vi "Program list Selection.vi"(8 "error in":errorcluster, 9 "FeedBack Channel":string[](array[string])=["fgdgfvcbc", "vnfhgjkn", "21354682"], 10 "Filepath":path=path "D:/My Project/2019-2020/Magnetic Mareli UM/MM_UM/Project Setup/data/program seq/Program_280A.bin", 11 "vi referenceIn":refnum<vi>) -> (0 "error out":errorcluster, 1 "Exit":bool, 2 "String":string, 3 "vi reference Out":refnum<vi>)   [LabVIEW 2015]
uses:
  Control Button/Exit.ctl
  Control Button/next.ctl
  Control Button/Control 11.ctl
  Galobal variable_TI.vi
  <vilib>/addons/database/Connection.llb/DB Tools Open Connec (String).vi
  <vilib>/addons/database/_DB Variant To Data/Database Variant To Data.xnode
  <vilib>/addons/database/NI_Database_API.lvlib
panel:
  out "error out 2":errorcluster
  out "String 2":string
  in  "Next":T1
  in  "Exit":T2
  in  "Program List":string(combo)
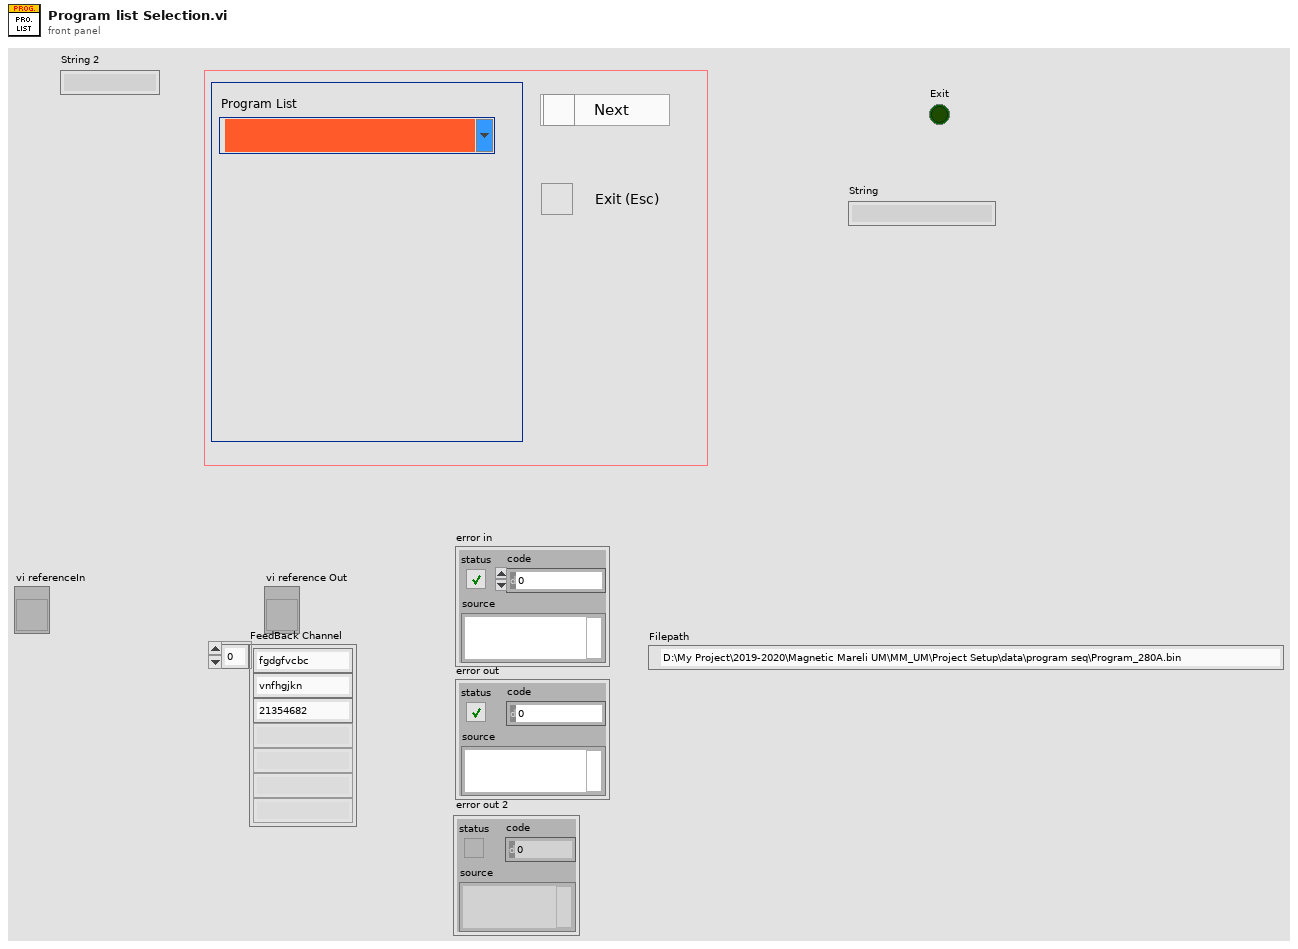
[diagram p1: front panel]
types:
  T1 = typedef "next.ctl" = bool
  T2 = typedef "Exit.ctl" = bool
  T3 = typedef "Control 11.ctl" = dbl
  T4 = enum32{"Invalid", "Standard", "Closed", "Hidden", "Minimized", "Maximized"}
  T5 = typedef "NI_Database_API.lvlib/Conn ObjectReference.ctl" = refnum<k1>
  T6 = cluster{"LVDT1Max AI0":dbl, "LVDT1Min AI0":dbl, "LVDT2Max AI1":dbl, "LVDT2Min AI1":dbl, "LVDT3Max AI2":dbl, "LVDT3Min AI2":dbl, "LVDT4Max AI3":dbl, "LVDT4Min AI3":dbl, "Model":string, "MIC Code":string}
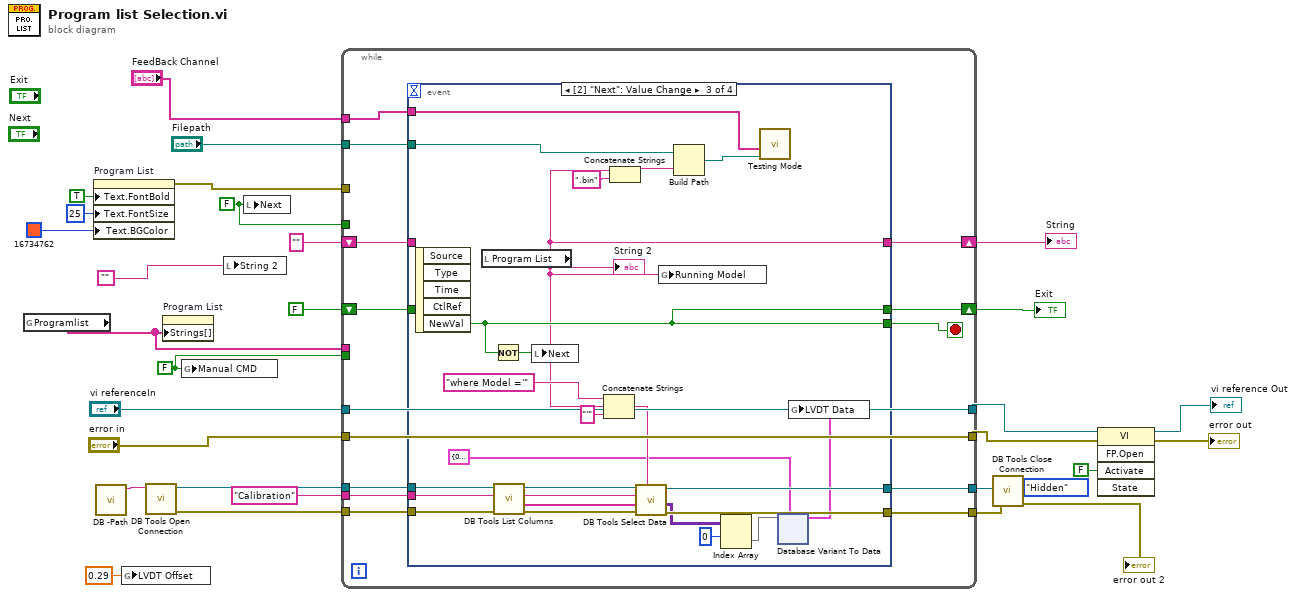
[diagram p0: block diagram]
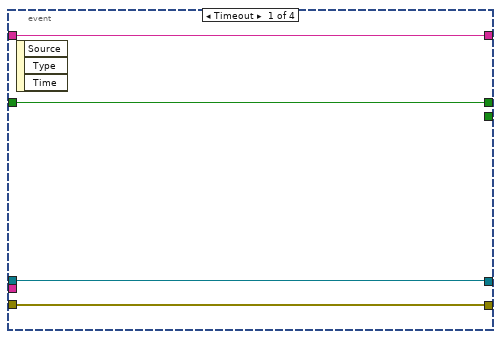
[diagram p2: hidden frame]
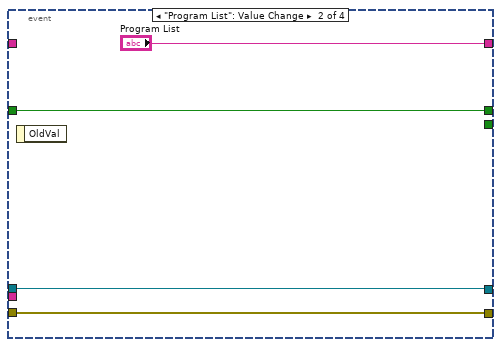
[diagram p3: hidden frame]
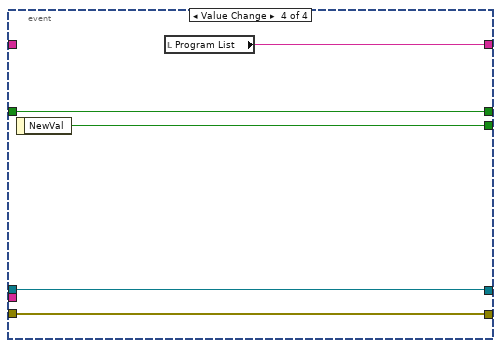
[diagram p4: hidden frame]
diagram:
  (unwired) T4."Hidden" ("State")
  w18 = FALSE ("Manual CMD")
  w19 = FALSE ("Next")
  n1 = global read "Galobal variable_TI.vi" "Programlist"() -> (w25:string[])
  n2 = property on="Program List" class="CmbBox"("Text.FontBold"=TRUE ("Text.Font:Bold"), "Text.FontSize"=u32 25 ("Text.Font:Size"), "Text.BGColor"=u32 16734762 ("Color Box")) -> (error out=w22:errorcluster)  [unwired: 2 in, 1 out]
  n3 = call "DB -Path.vi"() -> ("String"=w8:string)  [unwired: 11 in]
  n4 = global write "Galobal variable_TI.vi" "LVDT Offset"(T3 0.29 ("LVDT Offset")) -> ()
  n5 = call-poly <vilib>:"DB Tools Open Connection.vi"("connection information"=w8) -> ("error out"=w6:errorcluster, "connection reference"=w7:T5)  [unwired: 7 in]
  n6 = property on="Program List" class="CmbBox"("Strings[]"=w25) -> ()  [unwired: 2 in, 2 out]
  n7 = global write "Galobal variable_TI.vi" "Manual CMD"(w18) -> ()
  n8 = local write "String 2"("") -> ()
  n9 = local write "Next"(w19) -> ()
  n10 = while {
    shift-right: [w43] -> w29
    shift-left: "" ("Combo Box") -> [w42]
    shift-right: [w40] -> w26
    shift-left: T2 FALSE ("NewVal") -> [w39]
    tunnel: w25 -> [_]
    tunnel: w22 -> [_]
    tunnel: w19 -> [_]
    tunnel: w18 -> [_]
    tunnel: "vi referenceIn" -> [w38]
    tunnel: [w38] -> w12
    tunnel: "error in" -> [w37]
    tunnel: [w37] -> w11
    tunnel: "Filepath" -> [w36]
    tunnel: "FeedBack Channel" -> [w35]
    tunnel: w7 -> [w34]
    tunnel: w6 -> [w33]
    tunnel: "Calibration" ("table") -> [w32]
    tunnel: [w31] -> w4
    tunnel: [w30] -> w3
    stop <- w41 stop-if-true
    n11 = event shown="[2] \"Next\": Value Change" {
      selector: _ -> [_ _ _ _]
      dyn-events: _ -> [_ _ _ _]
      timeout: _ -> [_ _ _ _]
      tunnel: [w47 "Program List" w60 w393] -> w43
      tunnel: w42 -> [w47 _ _ _]
      tunnel: [_ _ w70 w394] -> w41
      tunnel: [w46 w50 w70 w392] -> w40
      tunnel: w39 -> [w46 w50 _ w392]
      tunnel: w36 -> [_ _ w73 _]
      tunnel: w35 -> [_ _ w71 _]
      tunnel: w34 -> [w45 w49 w66 w391]
      tunnel: w33 -> [w44 w48 w65 w390]
      tunnel: w32 -> [_ _ w63 _]
      tunnel: [w45 w49 w58 w391] -> w31
      tunnel: [w44 w48 w57 w390] -> w30
      event Timeout {
        n12 = event-data() -> ()  [unwired: 1 in, 3 out]
      }
      event "Program List": Value Change {
        n13 = event-data() -> ()  [unwired: 1 in, 1 out]
      }
      event Value Change {
        n14 = event-data() -> ("NewVal"=w70:T1)  [unwired: 1 in, 4 out]
        n15 = local read "Program List"() -> (w60:string)
        "String 2" <- w60
        n16 = Not(x=w70) -> (.not. x?=w69:T1)
        n17 = call <vilib>:"DB Tools List Columns.vi"("error in (no error)"=w65, "table"=w63, "connection reference"=w66) -> ("error out"=w68:errorcluster, "columns"=w67:string[], "connection reference out"=w64:T5)  [unwired: 1 in, 1 out]
        n18 = local write "Next"(w69) -> ()
        n19 = Concatenate Strings("where Model ='", w60, "'" ("string")) -> (w59:string)
        n20 = Concatenate Strings(w60, ".bin" ("string")) -> (w74:string)
        n21 = call <vilib>:"DB Tools Select Data.vi"("condition"=w59, "error in (no error)"=w68, "columns"=w67, "table"=w63, "connection reference"=w64) -> ("error out"=w57:errorcluster, "data"=w54:variant[][], "connection reference out"=w58:T5)  [unwired: 1 in]
        n22 = global write "Galobal variable_TI.vi" "Running Model"(w60) -> ()
        n23 = Build Path(base path=w73, name or relative path=w74) -> (appended path=w72:path)
        n24 = Index Array(array=w54, index (row)=0) -> (element=w55:variant[])  [unwired: 1 in]
        n25 = call "Testing Mode.vi"("Filepath"=w72, "FeedBack Channel"=w71) -> ()  [unwired: 10 in]
        n26 = xnode "Database Variant To Data"("database variant"=w55, "type"=T6 {"LVDT1Max AI0"=0.0, "LVDT1Min AI0"=0.0, "LVDT2Max AI1"=0.0, "LVDT2Min AI1"=0.0, "LVDT3Max AI2"=0.0, "LVDT3Min AI2"=0.0, "LVDT4Max AI3"=0.0, "LVDT4Min AI3"=0.0, "Model"="", "MIC Code"=""} ("Sensor Setting Data 3")) -> ("data"=w52:T6)  [unwired: 1 in, 1 out]
        n27 = global write "Galobal variable_TI.vi" "LVDT Data"(w52) -> ()
      }
      event Value Change {
        n28 = event-data() -> ("NewVal"=w394:T2)  [unwired: 1 in]
        n29 = local read "Program List"() -> (w393:string)
      }
    }
  }
  "String" <- w29
  "Exit" <- w26
  n30 = call <vilib>:"DB Tools Close Connection.vi"("error in (no error)"=w3, "connection reference"=w4) -> ("error out"=→"error out 2":errorcluster)  [unwired: 5 in]
  n31 = invoke class="VI" method="FP.Open"(reference=w12, error in=w11, "Activate"=FALSE ("Activate?")) -> (reference out=→"vi reference Out":refnum<vi>, error out=→"error out":errorcluster)  [unwired: 2 in, 3 out]
